vi "GetWinUserName.vi"(8 "Error In":errorcluster) -> (0 "Error Out":errorcluster, 3 "Windows User Name":string)   [LabVIEW 2017, in "Client.lvlib" / "CommsFrameWork.lvlib"]
uses:
  CommsFrameWork.lvlib
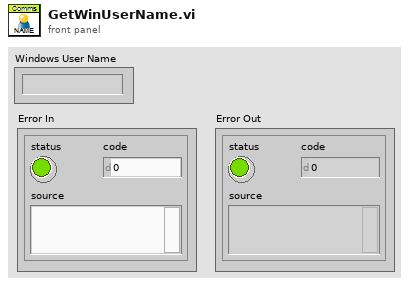
[diagram p1: front panel]
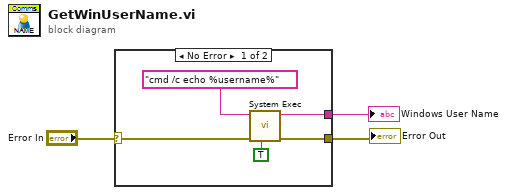
[diagram p0: block diagram]
diagram:
  n1 = case shown="No Error" "Error In" {
    selector: "Error In" -> [w6 w9]
    tunnel: [w8 _] -> w3
    tunnel: [w5 w9] -> w1
    frame No Error {
      n2 = call "System Exec.vi"("run minimized? (F)"=TRUE, "error in (no error)"=w6, "command line"="cmd /c echo %username%") -> ("error out"=w5:errorcluster, "standard output"=w8:string)  [unwired: 5 in, 2 out]
    }
    frame Error {
    }
  }
  "Windows User Name" <- w3
  "Error Out" <- w1
